vi "insert.vi"(5 "replace entry if exists (F)":bool, 6 "call chain index (1)":i32=1, 7 "vi ref (caller)":refnum<vi>, 8 "error in (no error)":errorcluster, 11 "entry":T1) -> (0 "error out":errorcluster)   [LabVIEW 2024, in "status manager.lvlib"]
uses:
  status manager.lvlib
  entry type.ctl
  insert or remove.ctl
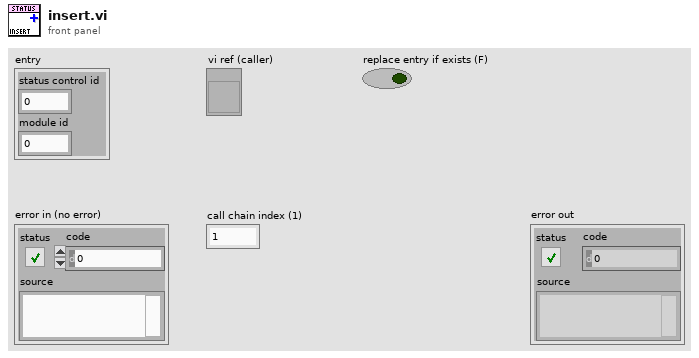
[diagram p1: front panel]
types:
  T1 = typedef "status manager.lvlib/entry type.ctl" = cluster{"status control id":i32, "module id":i32}
  T2 = typedef "status manager.lvlib/insert or remove.ctl" = enum16{"insert", "remove"}
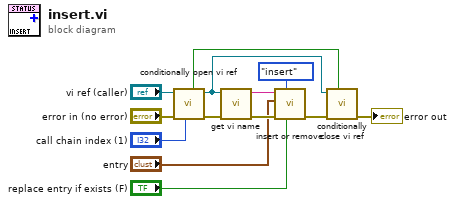
[diagram p0: block diagram]
diagram:
  n1 = call "conditionally open vi ref.vi"("call chain index (1)"="call chain index (1)", "error in (no error)"="error in (no error)", "vi ref in"="vi ref (caller)") -> ("error out"=w11:errorcluster, "vi ref out"=w5:refnum<vi>, "new ref?"=w4:bool)  [unwired: 6 in]
  n2 = call "get vi name.vi"("error in (no error)"=w11, "vi ref"=w5) -> ("error out"=w9:errorcluster, "vi name"=w10:string)  [unwired: 8 in]
  n3 = call "insert or remove.vi"("replace entry if exists"="replace entry if exists (F)", "action"=insert_or_remove."insert", "error in (no error)"=w9, "entry"="entry", "id"=w10) -> ("error out"=w8:errorcluster)  [unwired: 6 in]
  n4 = call "conditionally close vi ref.vi"("new ref?"=w4, "error in (no error)"=w8, "vi ref"=w5) -> ("error out"=→"error out":errorcluster)  [unwired: 8 in]
